vi "Dispose Images.vi"(0 "raw display notifier":refnum<notifier>, 11 "error in (no error)":errorcluster) -> (15 "error out":errorcluster)   [LabVIEW 2023, in "GettingStarted_Common_148X_Host.lvlib"]
uses:
  GettingStarted_Common_148X_Host.lvlib
  Types/Serial Channel Display Parameters.ctl
  <vilib>/vision/Image Controls.llb/IMAQ Image.ctl
  Types/RAW Interpretation for Display.ctl
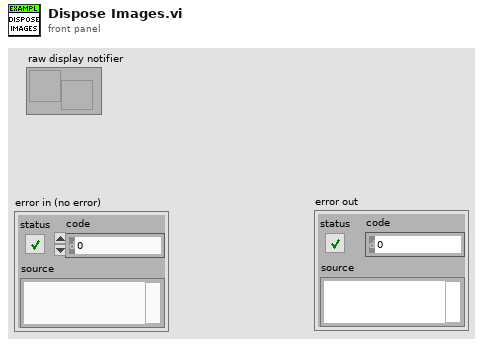
[diagram p1: front panel]
types:
  T1 = typedef "GettingStarted_Common_148X_Host.lvlib/Serial Channel Display Parameters.ctl" = cluster{"images":cluster{"grayscale":T2, "color":T2}, "RAW parameters":cluster{"interpretation":T3, "bayer parameters":cluster{"pattern":i32, "algorithm":i32, "red gain":dbl, "green gain":dbl, "blue gain":dbl}}}
  T2 = typedef "IMAQ Image.ctl" = refnum<image>
  T3 = typedef "GettingStarted_Common_148X_Host.lvlib/RAW Interpretation for Display.ctl" = enum16{"Grayscale", "Bayer", "RGB", "YUV422", "YUV420", "Legacy YUV420"}
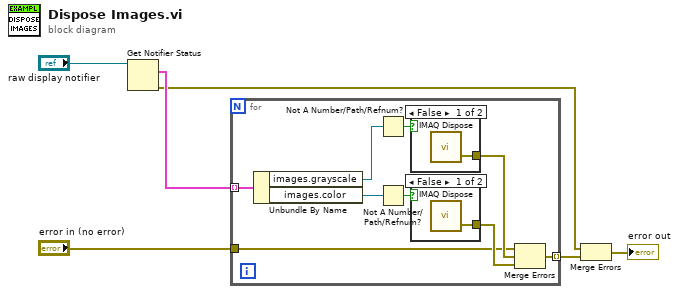
[diagram p0: block diagram]
diagram:
  n1 = Get Notifier Status(notifier="raw display notifier") -> (current notification=w2:T1[], error out=w1:errorcluster)  [unwired: 1 in, 3 out]
  n2 = for {
    tunnel: w2 -> [w14] mode=indexing
    tunnel: "error in (no error)" -> [w7]
    tunnel: [w8] -> w5 mode=indexing
    n3 = Unbundle By Name(w14) -> ("images.grayscale"=w10:T2, "images.color"=w13:T2)
    n4 = Not A Number/Path/Refnum?(number/path/refnum=w10) -> (NaN/Path/Refnum?=w11:bool)
    n5 = Not A Number/Path/Refnum?(number/path/refnum=w13) -> (NaN/Path/Refnum?=w15:bool)
    n6 = case shown="False" w11 {
      tunnel: [w16 _] -> w9
      frame False {
        n7 = call "IMAQ Dispose"() -> ("error out"=w16:errorcluster)  [unwired: 6 in]
      }
      frame True {
      }
    }
    n8 = case shown="False" w15 {
      tunnel: [w17 _] -> w12
      frame False {
        n9 = call "IMAQ Dispose"() -> ("error out"=w17:errorcluster)  [unwired: 6 in]
      }
      frame True {
      }
    }
    n10 = Merge Errors(w7, w9, w12) -> (w8:errorcluster)
  }
  n11 = Merge Errors(w1, w5) -> (→"error out":errorcluster)
